vi "ITX to LV 2.1 1D.vi"(8 "error in":errorcluster, 11 "file (use dialog)":path=path "P:/sample/GaAs/GaAs quantum dots/2008/PL Map/A1 735/060731ASBA_A1_6.0.itx") -> (0 "error out":errorcluster, 2 "1D arrays":dbl[][](array[numeric]), 3 "Data (Dictionary)":T1[](array[typedef]), 4 "Notes":string, 5 "base wavenames":string[](array[string]), 6 "Commands":string)   [LabVIEW 2016, in "LV to ITX.lvclass"]
uses:
  LV to ITX.lvclass
  Typedefs/Dictionary--cluster.ctl
panel:
  out "wavenames":string[](array[string])
  out "text to data":u32
  out "parse 2":u32
  out "parse 1 (ms)":u32
  out "open file (ms)":u32
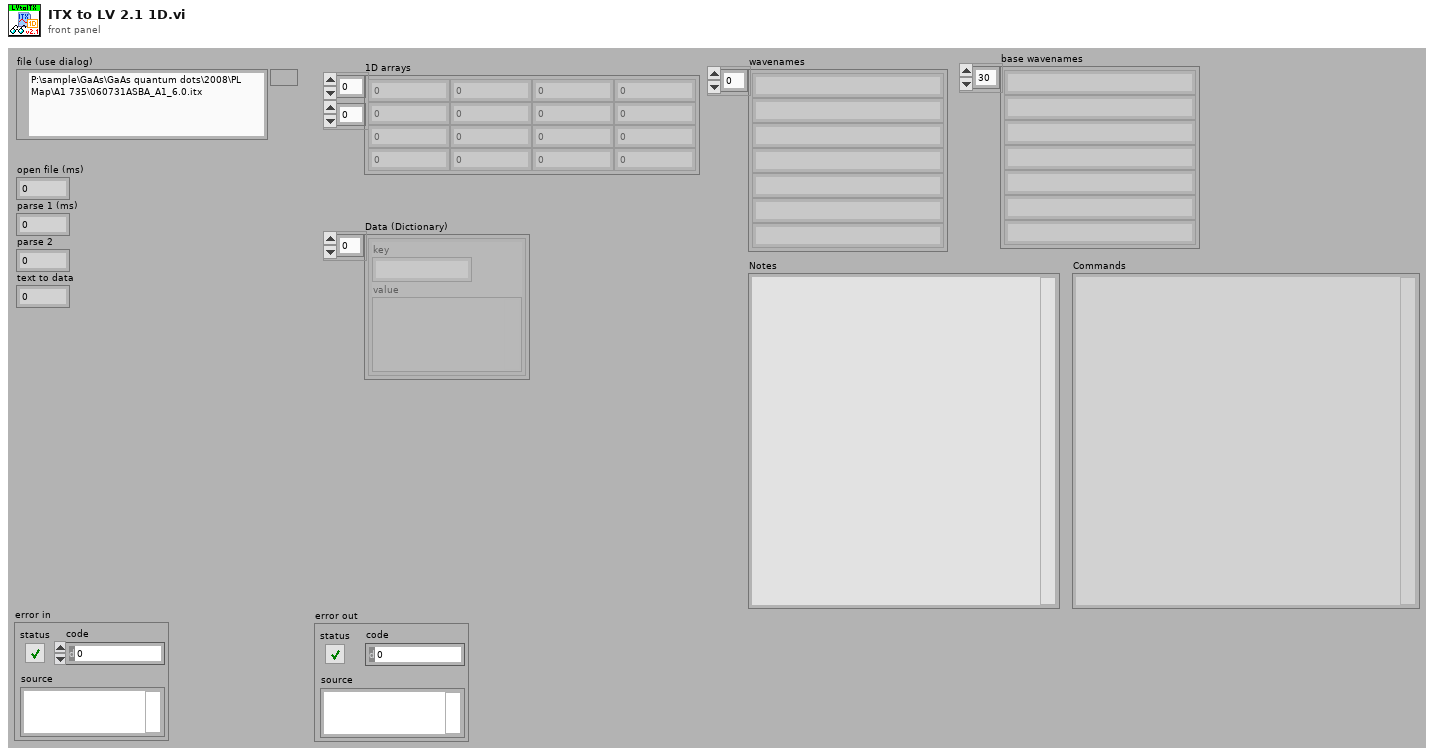
[diagram p1: front panel]
types:
  T1 = typedef "LV to ITX.lvclass/Dictionary--cluster.ctl" = cluster{"key":string, "value":variant}
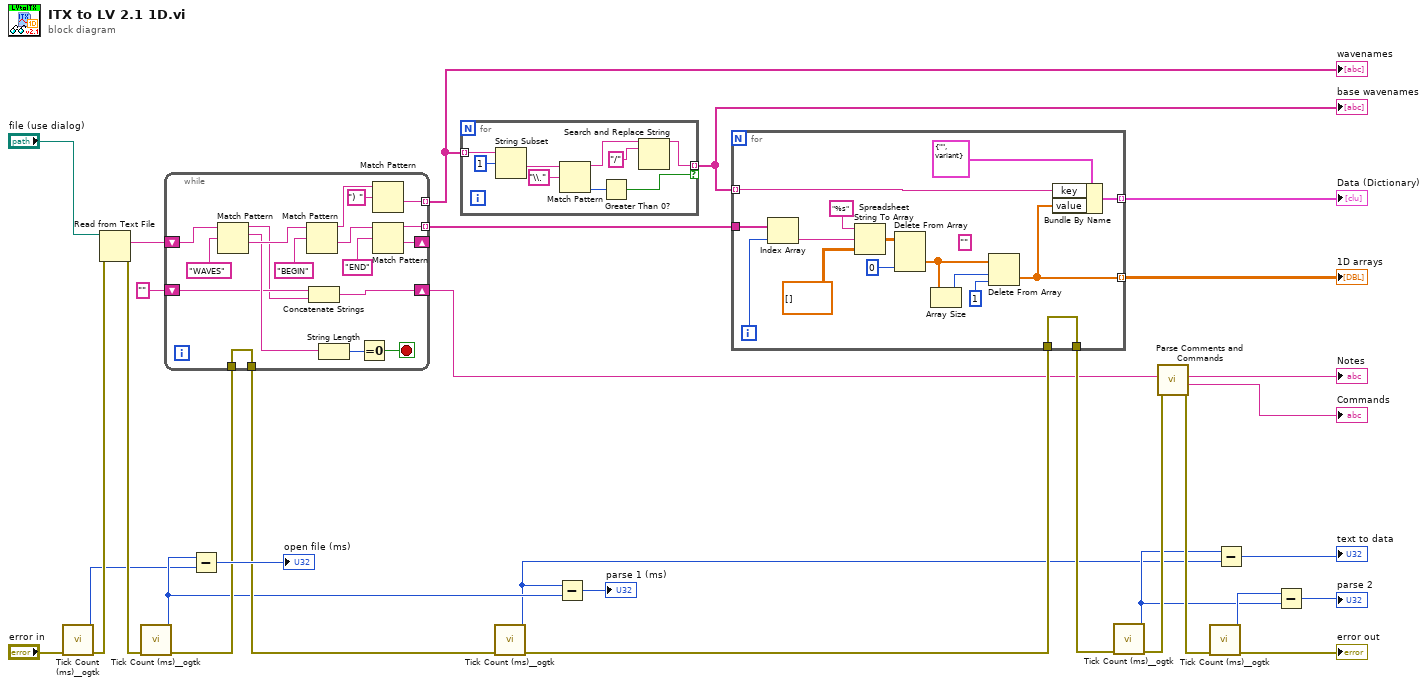
[diagram p0: block diagram]
diagram:
  n1 = call <userlib>:"Tick Count (ms)__ogtk.vi"("error in (no error)"="error in") -> ("error out"=w25:errorcluster, "millisecond timer value"=w2:u32)  [unwired: 9 in]
  n2 = Read from Text File(file (use dialog)="file (use dialog)", error in=w25) -> (text=w30:string, error out=w24:errorcluster)  [unwired: 1 in, 3 out]
  n3 = call <userlib>:"Tick Count (ms)__ogtk.vi"("error in (no error)"=w24) -> ("error out"=w17:errorcluster, "millisecond timer value"=w3:u32)  [unwired: 9 in]
  n4 = while {
    tunnel: [w32] -> w27 mode=indexing
    shift-right: [w46] -> _
    shift-left: w30 -> [w34]
    tunnel: [w42] -> w7 mode=indexing
    shift-right: [w37] -> w6
    shift-left: "" ("regular expression") -> [w36]
    tunnel: w17 -> [w31]
    tunnel: [w31] -> w11
    stop <- w43 stop-if-true
    n5 = Match Pattern(string=w34, regular expression="WAVES") -> (before substring=w35:string, match substring=w45:string, after substring=w48:string)  [unwired: 2 out]
    n6 = Match Pattern(string=w48, regular expression="BEGIN" ("regular expression 2")) -> (before substring=w33:string, after substring=w47:string)  [unwired: 3 out]
    n7 = Concatenate Strings(w36, w35) -> (w37:string)
    n8 = String Length(string=w45) -> (length=w44:i32)
    n9 = Equal To 0?(x=w44) -> (x = 0?=w43:bool)
    n10 = Match Pattern(string=w33, regular expression=") ") -> (after substring=w42:string)  [unwired: 4 out]
    n11 = Match Pattern(string=w47, regular expression="END" ("regular expression 3")) -> (before substring=w32:string, after substring=w46:string)  [unwired: 3 out]
  }
  "wavenames" <- w7
  n12 = Subtract(x=w3, y=w2) -> (x-y=→"open file (ms)":u32)
  n13 = for {
    tunnel: w7 -> [w56] mode=indexing
    tunnel: [w49] -> w8 mode=indexing if=w52
    n14 = String Subset(string=w56, offset (0)=1) -> (substring=w55:string)  [unwired: 1 in]
    n15 = Match Pattern(string=w55, regular expression="\\.") -> (before substring=w50:string, offset past match=w53:i32)  [unwired: 1 in, 2 out]
    n16 = Greater Than 0?(x=w53) -> (x > 0?=w52:bool)
    n17 = Search and Replace String(input string=w50, search string="/") -> (result string=w49:string)  [unwired: 6 in, 3 out]
  }
  "base wavenames" <- w8
  n18 = call <userlib>:"Tick Count (ms)__ogtk.vi"("error in (no error)"=w11) -> ("error out"=w16:errorcluster, "millisecond timer value"=w1:u32)  [unwired: 9 in]
  n19 = Subtract(x=w1, y=w3) -> (x-y=→"parse 1 (ms)":u32)
  n20 = for {
    tunnel: [w60] -> w29 mode=indexing
    tunnel: w27 -> [w67]
    tunnel: w16 -> [w62]
    tunnel: [w62] -> w12
    tunnel: w8 -> [w61] mode=indexing
    tunnel: [w59] -> w10 mode=indexing
    i -> [w64]
    (unwired) "" ("result string")
    n21 = Index Array(array=w67, index=w64) -> (element=w63:string)
    n22 = Spreadsheet String To Array(format string="%s", spreadsheet string=w63, array type (2D Dbl)=dbl[][] []) -> (array=w71:dbl[][])  [unwired: 1 out]
    n23 = Delete From Array(array=w71, index (col)=0 ("disabled index (col)")) -> (deleted portion=w70:dbl[])  [unwired: 2 in, 1 out]
    n24 = Array Size(array=w70) -> (size(s)=w69:i32)
    n25 = Delete From Array(array=w70, length=w69, index=1) -> (deleted portion=w60:dbl[])  [unwired: 1 out]
    n26 = Bundle By Name(cluster=T1 {"key"="", "value"=variant} ("key-value"), "key"=w61, "value"=w60) -> (w59:T1)
  }
  "1D arrays" <- w29
  "Data (Dictionary)" <- w10
  n27 = call <userlib>:"Tick Count (ms)__ogtk.vi"("error in (no error)"=w12) -> ("error out"=w20:errorcluster, "millisecond timer value"=w4:u32)  [unwired: 9 in]
  n28 = call "Parse Comments and Commands.vi"("error in"=w20, "Igor Comments and Commands"=w6) -> ("error out"=w13:errorcluster, "Commands"=→"Commands":string, "Comments"=→"Notes":string)  [unwired: 7 in]
  n29 = call <userlib>:"Tick Count (ms)__ogtk.vi"("error in (no error)"=w13) -> ("error out"=→"error out":errorcluster, "millisecond timer value"=w5:u32)  [unwired: 9 in]
  n30 = Subtract(x=w4, y=w1) -> (x-y=→"text to data":u32)
  n31 = Subtract(x=w5, y=w4) -> (x-y=→"parse 2":u32)
